vi "Vision - Get Current Image Filename.vi"(7 "Current Position":dbl, 8 "error in (no error)":errorcluster, 11 "Local Data":T1 {"Vision Settings"."Dist/Page" items=["Blue (M)/Black (C)", "Red (M)/Green (C)"]}) -> (0 "error out":errorcluster, 3 "Image Folder out":path)   [LabVIEW 2024]
uses:
  Controls/Vision - Local Data.ctl
  Controls/Test Cluster.ctl
  Controls/Excluded Information.ctl
  Controls/Language.ctl
  Controls/Device_Type.ctl
  <vilib>/Utility/miscctls.llb/LVRectTypeDef.ctl
  <vilib>/Utility/miscctls.llb/LVBoundsTypeDef.ctl
  Controls/Vision - Reporting Settings.ctl
  Controls/Vision - Dist Per Page.ctl
  Controls/Vision - Section.ctl
  Buttons/Bin.ctl
  Controls/Vision - Image Dimension Command.ctl
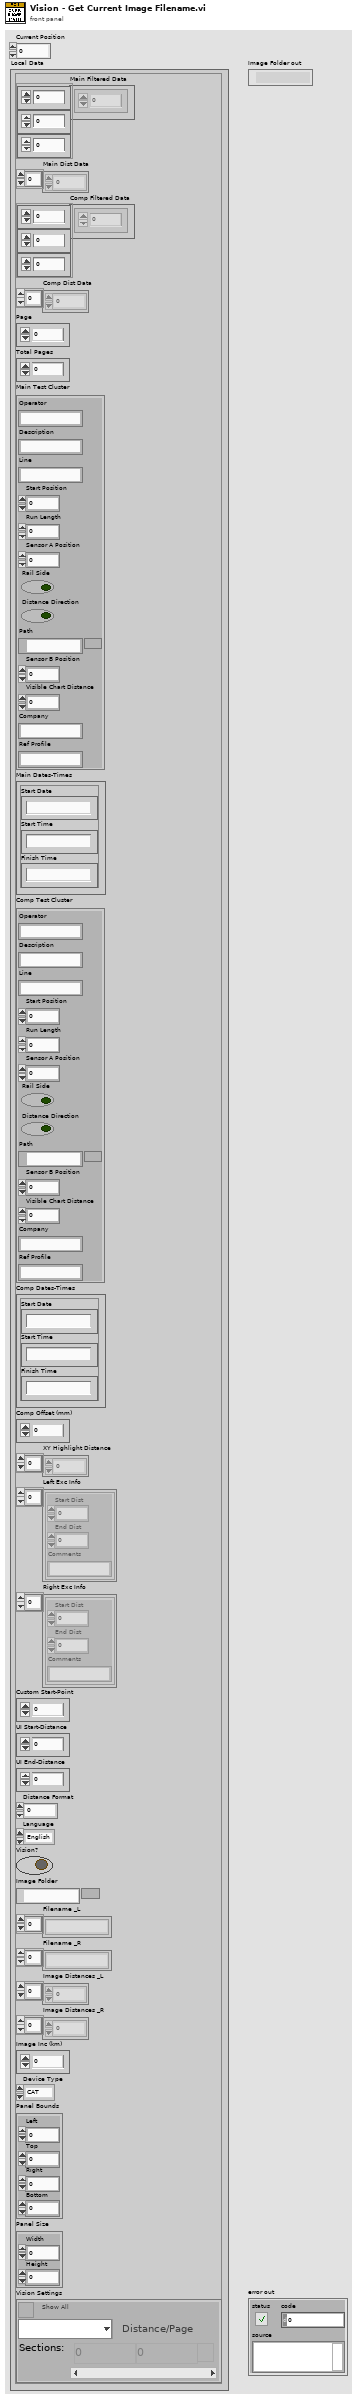
[diagram p1: front panel]
types:
  T1 = typedef "Vision - Local Data.ctl" = cluster{"Main Filtered Data":dbl[][][], "Main Dist Data":dbl[], "Comp Filtered Data":dbl[][][], "Comp Dist Data":dbl[], "Page":u8, "Total Pages":u8, "Main Test Cluster":T2, "Main Dates-Times":cluster{"Start Date":string, "Start Time":string, "Finish Time":string}, "Comp Test Cluster":T2, "Comp Dates-Times":cluster{"Start Date":string, "Start Time":string, "Finish Time":string}, "Comp Offset (mm)":i64, "XY Highlight Distance":dbl[], "Left Exc Info":T3[], "Right Exc Info":T3[], "Custom Start-Point":dbl, "UI Start-Distance":dbl, "UI End-Distance":dbl, "Distance Format":u8, "Language":T4, "Vision?":bool, "Image Folder":path, "Filename _L":string[], "Filename _R":string[], "Image Distances _L":dbl[], "Image Distances _R":dbl[], "Image Inc (km)":dbl, "Device Type":T5, "Panel Bounds":T6, "Panel Size":T7, "Vision Settings":T8}
  T2 = typedef "Test Cluster.ctl" = cluster{"Operator":string, "Description":string, "Line":string, "Start Position":dbl, "Run Length":dbl, "Sensor A Position":dbl, "Rail Side":bool, "Distance Direction":bool, "Path":path, "Sensor B Position":dbl, "Visible Chart Distance":dbl, "Company":string, "Ref Profile":string}
  T3 = typedef "Excluded Information.ctl" = cluster{"Start Dist":dbl, "End Dist":dbl, "Comments":string}
  T4 = typedef "Language.ctl" = enum16{"English", "Chinese", "German"}
  T5 = typedef "Device_Type.ctl" = enum16{"CAT", "Bi-CAT", "YRCA", "RCA", "RV-HR", "TV-HR"}
  T6 = typedef "LVRectTypeDef.ctl" = cluster{"Left":i16, "Top":i16, "Right":i16, "Bottom":i16}
  T7 = typedef "LVBoundsTypeDef.ctl" = cluster{"Width":u32, "Height":u32}
  T8 = typedef "Vision - Reporting Settings.ctl" = cluster{"Show All?":bool, "Dist/Page":T9, "Sections":T10[]}
  T9 = typedef "Vision - Dist Per Page.ctl" = u16
  T10 = typedef "Vision - Section.ctl" = cluster{"From":dbl, "To":dbl, "Discard":T11}
  T11 = typedef "Bin.ctl" = bool
  T12 = typedef "Vision - Image Dimension Command.ctl" = enum16{"Get All Dims", "Get # of Images"}
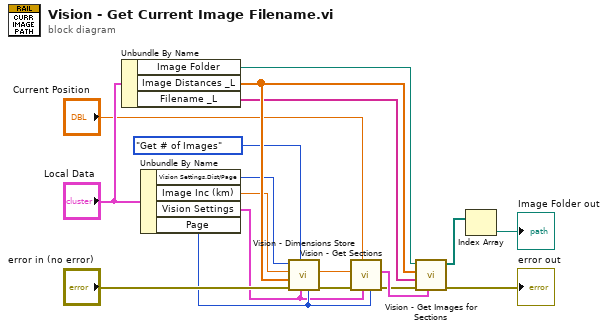
[diagram p0: block diagram]
diagram:
  n1 = Unbundle By Name("Local Data") -> ("Image Folder"=w2:path, "Image Distances _L"=w13:dbl[], "Filename _L"=w3:string[])
  n2 = Unbundle By Name("Local Data") -> ("Vision Settings.Dist/Page"=w6:T9, "Image Inc (km)"=w8:dbl, "Vision Settings"=w11:T8, "Page"=w12:u8)
  n3 = call "Vision - Dimensions Store.vi"("Page"=w12, "Supervisory Config Cluster In"=w11, "Command"=Vision_-_Image_Dimension_Command."Get # of Images", "error in (no error)"="error in (no error)", "Image Distances _L"=w13, "Inc/page (km)"=w8, "Dist/Page Index"=w6) -> ("error out"=w4:errorcluster, "Dist/Page (km)"=w10:dbl)  [unwired: 1 in, 2 out]
  n4 = call "Vision - Get Sections.vi"("Page"=w12, "Supervisory Config Cluster In"=w11, "Current Pos (km)"="Current Position", "error in (no error)"=w4, "Inc/page (km)"=w10) -> ("error out"=w7:errorcluster, "Sections Out"=w9:T10[])  [unwired: 5 in]
  n5 = call "Vision - Get Images for Sections.vi"("Sections"=w9, "error in (no error)"=w7, "Filename _L"=w3, "Image Distances _L"=w13, "Image Folder in"=w2) -> ("error out"=→"error out":errorcluster, "Image Paths"=w17:path[])  [unwired: 4 in, 1 out]
  n6 = Index Array(array=w17) -> (element=→"Image Folder out":path)  [unwired: 1 in]
